vi "LVVersionCheck_Global_Init.vi"(11 "Object":T1) -> ()   [LabVIEW 2015]
doc: "#translatableVI"
uses:
  <resource>/Framework/Providers/API/ItemRef.ctl
  <resource>/Framework/Providers/API/mxLvMenuItem.ctl
  LV Project Version Check.lvlib
panel:
  out "error out":errorcluster
  in  "error in":errorcluster
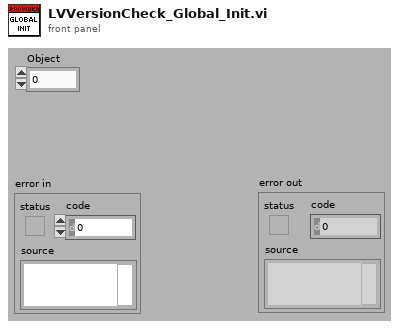
[diagram p1: front panel]
types:
  T1 = typedef "ItemRef.ctl" = u64
  T2 = typedef "mxLvMenuItem.ctl" = cluster{"Menu Name":string, "Description":string, "Icon File Name":path, "Menu Tag":string, "Enabled":bool, "Checked":bool, "Separator":bool, "Batchable":bool, "Weight":i32, "Batch Mode (Ignored if Not Batchable)":enum32{"Show If All Items Support Command", "Show If Any Items Support Command"}, "Menu Location":enum32{"<None>", "Project", "Project / Build Specifications", "Tools", "Tools / Source Control", "Tools / Real-Time Module", "Help"}, "Exclude From Getting Started Window Menu":bool}
  T3 = enum32{"<None>", "Project", "Project / Build Specifications", "Tools", "Tools / Source Control", "Tools / Real-Time Module", "Help"}
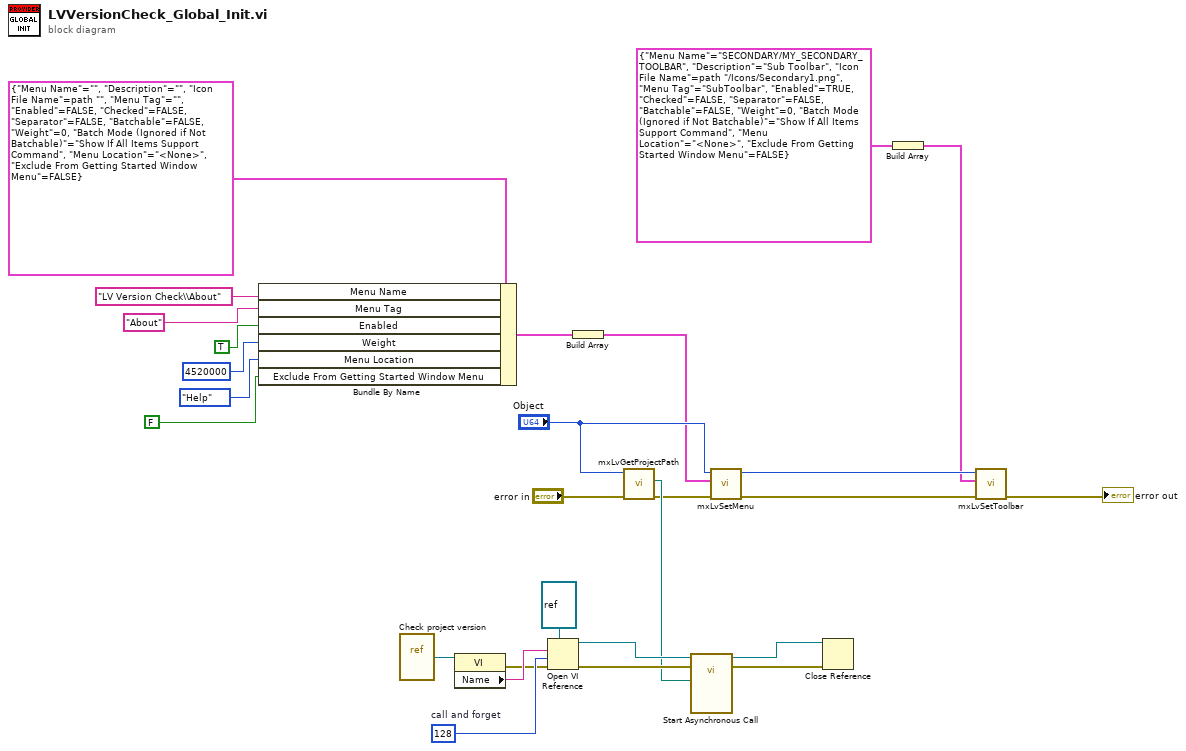
[diagram p0: block diagram]
diagram:
  w26 = 128  # call and forget
  n1 = Bundle By Name(cluster=T2 {"Menu Name"="", "Description"="", "Icon File Name"=path "", "Menu Tag"="", "Enabled"=FALSE, "Checked"=FALSE, "Separator"=FALSE, "Batchable"=FALSE, "Weight"=0, "Batch Mode (Ignored if Not Batchable)"=enum."Show If All Items Support Command", "Menu Location"=enum."<None>", "Exclude From Getting Started Window Menu"=FALSE} ("Menu Item"), "Menu Name"="LV Version Check\\About" ("element"), "Menu Tag"="About" ("menu tag"), "Enabled"=TRUE ("Checked"), "Weight"=4520000 ("menu weight"), "Menu Location"=T3."Help", "Exclude From Getting Started Window Menu"=FALSE) -> (w2:T2)
  n2 = vi-ref "Check project version.vi"() -> (w20:refnum<vi>)
  n3 = property class="VI"(reference=w20) -> (error out=w18:errorcluster, "Name"=w19:string)  [unwired: 1 in, 1 out]
  n4 = Open VI Reference(type specifier VI Refnum (for type only)=refnum<vi> refnum, vi path=w19, options=w26, error in (no error)=w18) -> (vi reference=w24:refnum<vi>, error out=w23:errorcluster)  [unwired: 2 in]
  n5 = Build Array(w2) -> (w1:T2[])
  n6 = call <resource>:"mxLvGetProjectPath.vi"("error in"="error in", "Item"="Object") -> ("error out"=w14:errorcluster, "Project Path"=w17:path)  [unwired: 7 in, 1 out]
  n7 = call-by-ref "Start Asynchronous Call"(reference=w24, error in=w23, "path to XML document"=w17) -> (reference out=w21:refnum<vi>, error out=w22:errorcluster)  [unwired: 11 in]
  n8 = call <resource>:"mxLvSetMenu.vi"("error in"=w14, "Menu Items"=w1, "Item"="Object") -> ("error out"=w15:errorcluster, "Item"=w16:T1)  [unwired: 7 out]
  n9 = Close Reference(reference=w21, error in (no error)=w22) -> ()  [unwired: 1 out]
  n10 = Build Array(T2 {"Menu Name"="SECONDARY/MY_SECONDARY_TOOLBAR", "Description"="Sub Toolbar", "Icon File Name"=path "../Icons/Secondary1.png", "Menu Tag"="SubToolbar", "Enabled"=TRUE, "Checked"=FALSE, "Separator"=FALSE, "Batchable"=FALSE, "Weight"=0, "Batch Mode (Ignored if Not Batchable)"=enum."Show If All Items Support Command", "Menu Location"=enum."<None>", "Exclude From Getting Started Window Menu"=FALSE} ("Menu Item")) -> (w10:T2[])
  n11 = call <resource>:"mxLvSetToolbar.vi"("error in"=w15, "Toolbar Items"=w10, "Item"=w16) -> ("error out"=→"error out":errorcluster)  [unwired: 7 in, 1 out]
